vi "Autonomous Independent.vi"() -> ()   [LabVIEW 2013]
doc: "This VI is called when autonomous begins, and will automatically be terminated when autonomous ends. You can carry out timed or sensor driven robot movement independently without needing to return to the caller."
uses:
  <vilib>/Rock Robotics/WPI/Solenoid/WPI_SolenoidValue.ctl
  Robot Global Data.vi
  <vilib>/Rock Robotics/WPI/Solenoid/WPI_SolenoidSetEnum.vi
  <vilib>/Rock Robotics/WPI/RobotDrive/WPI_RobotDriveArcadeDrive_Standard(NoSaturation).vi
  <vilib>/Rock Robotics/WPI/RobotDrive/WPI_RobotDriveGetSetRefNum.vi
  <vilib>/Rock Robotics/WPI/Joystick/WPI_JoystickGetSetRefNum.vi
panel:
  in  "Current Shooter Status":T1(ring)=enum."Ready to fire"
  out "Timer for firing mech":dbl
  out "Hot?":bool
  out "Current Movement, for debugging":T2 {"Y Joystick Value" scale=1.0..-1.0; "X Joystick Value" scale=-1.0..1.0}
  in  "Array of robot movements":T3(array[cluster]) {"Y Joystick Value" scale=1.0..-1.0; "X Joystick Value" scale=-1.0..1.0}
  # "Be sure to right-click and choose Data Operations>>Make Current Value default if you want to save the array values with the VI"
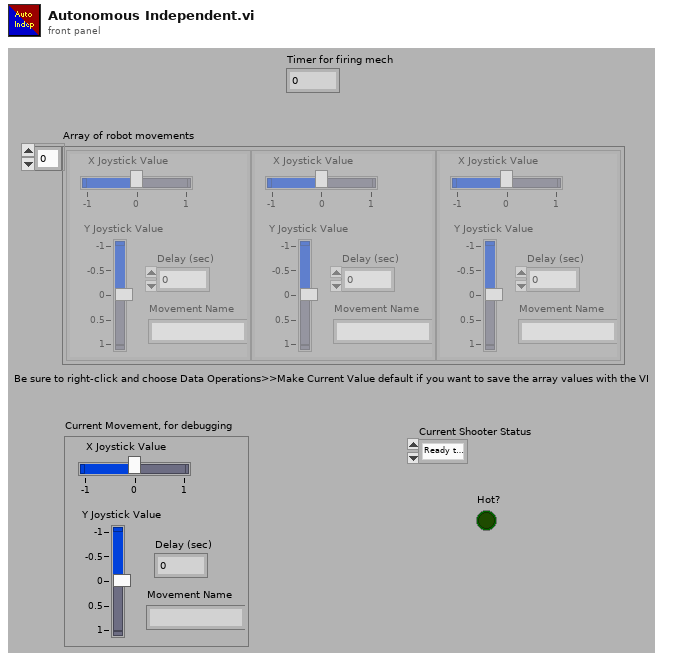
[diagram p1: front panel]
types:
  T1 = enum16{"Retracting", "Firing", "Ready to fire", "Pulling back", "Just fired"}
  T2 = cluster{"X Joystick Value":dbl, "Y Joystick Value":dbl, "Delay (sec)":dbl, "Movement Name":string}
  T3 = cluster{"X Joystick Value":dbl, "Y Joystick Value":dbl, "Delay (sec)":dbl, "Movement Name":string}[]
  T4 = typedef "WPI_JoystickDevRef.ctl" = cluster{"Device":T5}
  T5 = typedef "WPI_JoystickDeviceEnum.ctl" = enum16{"USB 1", "USB 2", "USB 3", "USB 4", "Kinect 1", "Kinect 2"}
  T6 = cluster{"axis 1 (x)":dbl, "axis 2 (y)":dbl, "axis 3 (throttle)":dbl, "axis 4":dbl, "axis 5":dbl, "axis 6":dbl}
  T7 = typedef "WPI_MotorControlDeviceRef.ctl" = cluster{"DeviceStatus":errorcluster, "Type":enum16{"PWM", "CAN"}, "PWM":cluster{"Digital Module":T8, "PWM Channel":T9, "DeadBand":T10}, "CAN":cluster{"Device Number":u8, "Control Mode":T11, "Semaphore":T12, "Max Vout":dbl}, "Invert":bool, "TransformRef":T13, "InvTransformRef":T13}
  T8 = typedef "FPGA_TypedefDigitalModule.ctl" = enum16{"Digital Module 1", "Digital Module 2"}
  T9 = typedef "FPGA_DIOPWMChannel.ctl" = enum8{"PWM 1", "PWM 2", "PWM 3", "PWM 4", "PWM 5", "PWM 6", "PWM 7", "PWM 8", "PWM 9", "PWM 10", "Invalid"}
  T10 = typedef "WPI_PWMDeadband.ctl" = cluster{"Name":string, "maxPositivePwm":i32, "minPositivePwm":i32, "centerPwm":i32, "maxNegativePwm":i32, "minNegativePwm":i32, "angularRange":u16}
  T11 = typedef "WPI_CANJaguar_ControlMode.ctl" = enum8{"Percent VBus", "Current", "Speed", "Position", "Voltage"}
  T12 = typedef "Semaphore RefNum" = refnum<k1>
  T13 = typedef "WPI_PWMTransform_ConPane.ctl" = refnum<vi>
  T14 = typedef "WPI_RobotDriveDevRef.ctl" = cluster{"DevStatus":errorcluster, "Motors[]":T7[], "Square Inputs":bool, "Max Output":dbl, "Isochronous":bool}
  T15 = typedef "WPI_EncoderDevRef.ctl" = cluster{"DevStatus":errorcluster, "EncoderIndex":T16, "CounterIndex":T17, "DistancePerCount":dbl, "Decoding Type":T18}
  T16 = typedef "FPGA_EncoderIdx.ctl" = enum8{"Enc 0", "Enc 1", "Enc 2", "Enc 3", "Invalid"}
  T17 = typedef "FPGA_CounterCtrSystemIndex.ctl" = enum8{"Ctr 0", "Ctr 1", "Ctr 2", "Ctr 3", "Ctr 4", "Ctr 5", "Ctr 6", "Ctr 7", "Invalid"}
  T18 = typedef "WPI_EncoderType.ctl" = enum16{"1x", "2x", "4x"}
  T19 = typedef "WPI_DigitalInputDevRef.ctl" = cluster{"DevStatus":errorcluster, "DIO Channel":T20, "Digital Module":T8}
  T20 = typedef "FPGA_DIOChannel.ctl" = enum8{"DIO 1", "DIO 2", "DIO 3", "DIO 4", "DIO 5", "DIO 6", "DIO 7", "DIO 8", "DIO 9", "DIO 10", "DIO 11", "DIO 12", "DIO 13", "DIO 14", "Invalid"}
  T21 = typedef "WPI_SolenoidValue.ctl" = enum16{"Off", "On", "Forward", "Reverse"}
  T22 = typedef "WPI_SolenoidDevRef.ctl" = cluster{"DevStatus":errorcluster, "Solenoid Module":T23, "Forward Solenoid Channel":T24, "Reverse Solenoid Channel":T24}
  T23 = typedef "FPGA_TypedefSolenoidModule.ctl" = enum16{"Solenoid Module 1", "Solenoid Module 2"}
  T24 = typedef "WPI_SolenoidChannel.ctl" = enum8{"Solenoid 1", "Solenoid 2", "Solenoid 3", "Solenoid 4", "Solenoid 5", "Solenoid 6", "Solenoid 7", "Solenoid 8", "Invalid"}
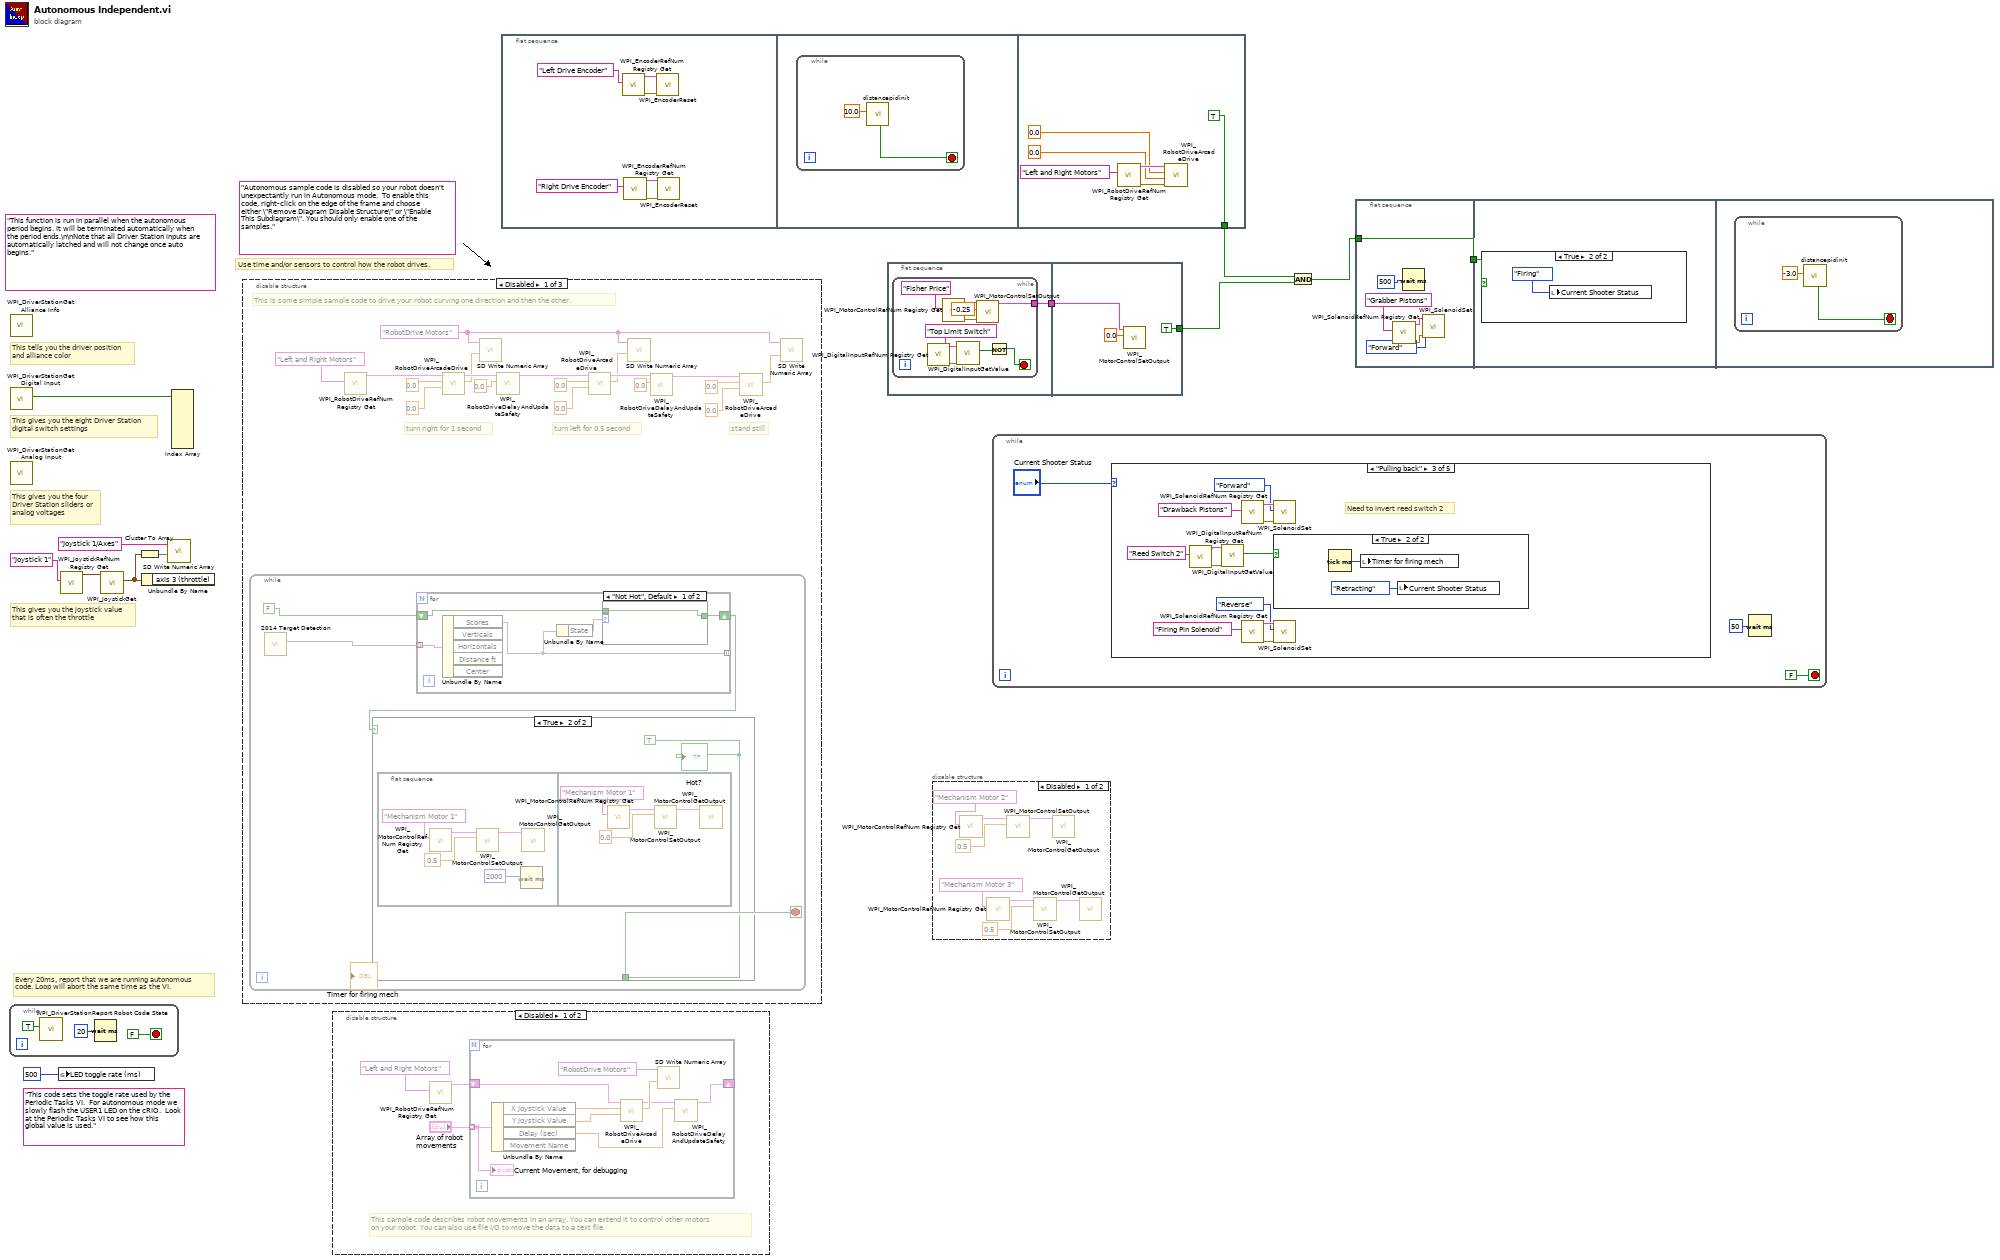
[diagram p0: block diagram]
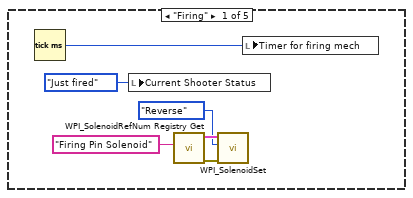
[diagram p3: hidden frame]
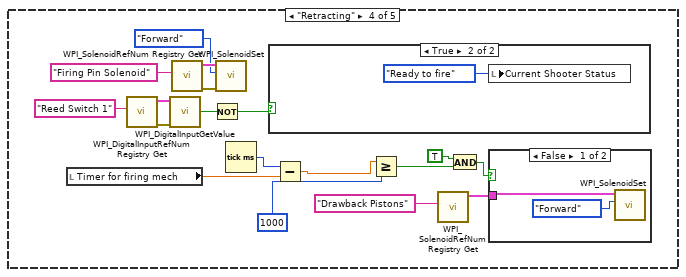
[diagram p6: hidden frame]
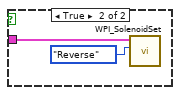
[diagram p8: hidden frame]
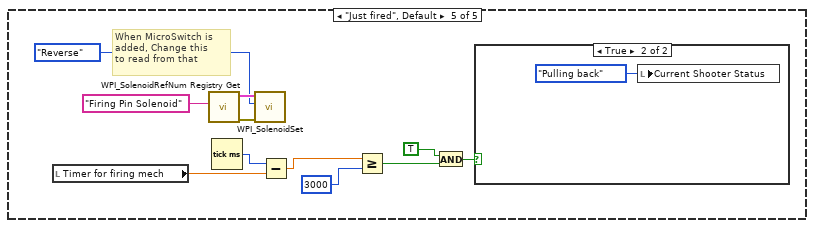
[diagram p9: hidden frame]
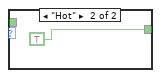
[diagram p13: hidden frame]
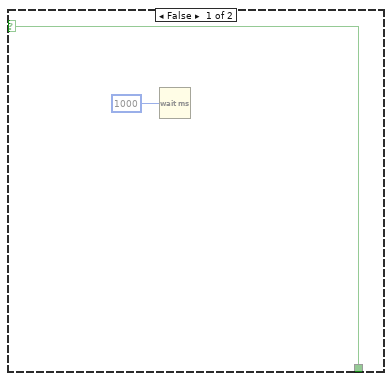
[diagram p14: hidden frame]
diagram:
  (unwired) "This code sets the toggle rate used by the Periodic Tasks VI.  For autonomous mode we slowly flash the USER1 LED on the cRIO.  Look at the Periodic Tasks VI to see how this global value is used."
  (unwired) "Autonomous sample code is disabled so your robot doesn't unexpectantly run in Autonomous mode.  To enable this code, right-click on the edge of the frame and choose either \"Remove Diagram Disable Structure\" or \"Enable This Subdiagram\". You should only enable one of the samples."
  (unwired) "This function is run in parallel when the autonomous period begins. It will be terminated automatically when the period ends.\n\nNote that all Driver Station inputs are automatically latched and will not change once auto begins."
  # "Every 20ms, report that we are running autonomous\ncode. Loop will abort the same time as the VI."
  # "This gives you the joystick value\nthat is often the throttle"
  # "Use time and/or sensors to control how the robot drives."
  # "This tells you the driver position\nand alliance color"
  # "This gives you the eight Driver Station\ndigital switch settings"
  # "This gives you the four\nDriver Station sliders or\nanalog voltages"
  n1 = while {
    stop <- FALSE stop-if-true
    n2 = call <vilib>:"WPI_DriverStationReport Robot Code State.vi"("Autonomous"=TRUE) -> ()  [unwired: 10 in, 1 out]
    n3 = Wait (ms)(milliseconds to wait=u32 20) -> ()  [unwired: 1 out]
  }
  n4 = call <vilib>:"WPI_DriverStationGet Alliance Info.vi"() -> ()  [unwired: 12 out]
  n5 = call <vilib>:"WPI_DriverStationGet Digital Input.vi"() -> ("Driver Station Digital Input (1-8)"=w12:bool[])  [unwired: 11 out]
  n6 = call <vilib>:"WPI_DriverStationGet Analog Input.vi"() -> ()  [unwired: 12 out]
  n7 = global write "Robot Global Data.vi" "LED toggle rate (ms)"(u32 500 ("LED ms toggle rate")) -> ()
  n8 = call <vilib>:"WPI_JoystickRefNum Registry Get.vi"("refnum name"="Joystick 1") -> ("JoystickDevRef"=w10:T4)  [unwired: 1 in, 9 out]
  n9 = call <vilib>:"WPI_JoystickGet.vi"("JoystickDevRef"=w10) -> ("Axes"=w7:T6)  [unwired: 1 in, 5 out]
  n10 = Cluster To Array(cluster=w7) -> (array=w8:dbl[])
  n11 = Unbundle By Name(w7) -> ()  [unwired: 1 out]
  n12 = call <vilib>:"SD Write Numeric Array.vi"("Numeric Array"=w8, "Name"="Joystick 1/Axes") -> ()  [unwired: 8 in, 2 out]
  n13 = Index Array(array=w12) -> ()  [unwired: 8 in, 8 out]
  n14 = disable-structure shown="Disabled" {
    frame Disabled {
      w16 = "RobotDrive Motors" ("Name")
      # "This is some simple sample code to drive your robot curving one direction and then the other."
      # "stand still"
      # "turn left for 0.5 second"
      # "turn right for 1 second"
      n15 = while {
        stop <- w37 stop-if-true
        n16 = call "2014 Target Detection.vi"() -> (2:w36)  [unwired: 11 in]
        n17 = for {
          tunnel: w36 -> [w42] mode=indexing
          tunnel: [w41] -> _ mode=indexing
          shift-right: [w39] -> w34
          shift-left: FALSE -> [w38]
          n18 = Unbundle By Name(w42) -> ("Scores"=w41)  [unwired: 4 out]
          n19 = Unbundle By Name(w41) -> ("State"=w40)
          n20 = case shown="\"Not Hot\", Default" w40 {
            tunnel: [w43 TRUE] -> w39
            tunnel: w38 -> [w43 _]
            frame "Not Hot", Default {
            }
            frame "Hot" {
            }
          }
        }
        n21 = case shown="True" w34 {
          selector: w34 -> [w45 _]
          tunnel: [w45 w47] -> w37
          frame False {
            n22 = Wait (ms)(milliseconds to wait=1000) -> ()  [unwired: 1 out]
          }
          frame True {
            w47 = TRUE
            n23 = flat-sequence {
              frame #0 {
                n24 = call <vilib>:"WPI_MotorControlRefNum Registry Get.vi"("refnum name"="Mechanism Motor 1") -> ("MotorControlDevRef"=w51:T7)  [unwired: 9 in, 1 out]
                n25 = call <vilib>:"WPI_MotorControlSetOutput.vi"("Output"=0.5, "MotorControlDevRef"=w51) -> ("MotorControlDevRef"=w49:T7)  [unwired: 7 in, 2 out]
                n26 = Wait (ms)(milliseconds to wait=2000) -> ()  [unwired: 1 out]
                n27 = call <vilib>:"WPI_MotorControlGetOutput.vi"("MotorControlDevRef"=w49) -> ()  [unwired: 8 in, 3 out]
              }
              frame #1 {
                n28 = call <vilib>:"WPI_MotorControlRefNum Registry Get.vi"("refnum name"="Mechanism Motor 1") -> ("MotorControlDevRef"=w55:T7)  [unwired: 9 in, 1 out]
                n29 = call <vilib>:"WPI_MotorControlSetOutput.vi"("Output"=0.0, "MotorControlDevRef"=w55) -> ("MotorControlDevRef"=w53:T7)  [unwired: 7 in, 2 out]
                n30 = call <vilib>:"WPI_MotorControlGetOutput.vi"("MotorControlDevRef"=w53) -> ()  [unwired: 8 in, 3 out]
              }
            }
            "Hot?" <- w47
          }
        }
      }
      n31 = call <vilib>:"WPI_RobotDriveRefNum Registry Get.vi"("refnum name"="Left and Right Motors") -> ("RobotDriveDevRef"=w20:T14)  [unwired: 1 in, 9 out]
      n32 = call-poly <vilib>:"WPI_RobotDriveArcadeDrive.vi"("Y axis value"=0.0 ("X axis value"), "X axis value"=0.0, "RobotDriveDevRef"=w20) -> ("Motor Values"=w19:dbl[], "RobotDriveDevRef"=w27:T14)  [unwired: 1 in, 6 out]
      n33 = call <vilib>:"SD Write Numeric Array.vi"("Numeric Array"=w19, "Name"=w16) -> ()  [unwired: 8 in, 2 out]
      n34 = call <vilib>:"WPI_RobotDriveDelayAndUpdateSafety.vi"("Delay (s)"=0.0, "RobotDriveDevRef"=w27) -> ("RobotDriveDevRef 2"=w26:T14)  [unwired: 8 in, 1 out]
      n35 = call-poly <vilib>:"WPI_RobotDriveArcadeDrive.vi"("Y axis value"=0.0 ("X axis value"), "X axis value"=0.0, "RobotDriveDevRef"=w26) -> ("Motor Values"=w18:dbl[], "RobotDriveDevRef"=w25:T14)  [unwired: 1 in, 6 out]
      n36 = call <vilib>:"SD Write Numeric Array.vi"("Numeric Array"=w18, "Name"=w16) -> ()  [unwired: 8 in, 2 out]
      n37 = call <vilib>:"WPI_RobotDriveDelayAndUpdateSafety.vi"("Delay (s)"=0.0, "RobotDriveDevRef"=w25) -> ("RobotDriveDevRef 2"=w24:T14)  [unwired: 8 in, 1 out]
      n38 = call-poly <vilib>:"WPI_RobotDriveArcadeDrive.vi"("Y axis value"=0.0 ("X axis value"), "X axis value"=0.0, "RobotDriveDevRef"=w24) -> ("Motor Values"=w17:dbl[])  [unwired: 1 in, 7 out]
      n39 = call <vilib>:"SD Write Numeric Array.vi"("Numeric Array"=w17, "Name"=w16) -> ()  [unwired: 8 in, 2 out]
    }
    frame Disabled {
    }
    frame Enabled {
    }
  }
  n40 = disable-structure shown="Disabled" {
    frame Disabled {
      # "This sample code describes robot movements in an array. You can extend it to control other motors\non your robot. You can also use file I/O to move the data to a text file."
      n41 = call <vilib>:"WPI_RobotDriveRefNum Registry Get.vi"("refnum name"="Left and Right Motors") -> ("RobotDriveDevRef"=w58:T14)  [unwired: 1 in, 9 out]
      n42 = for {
        shift-right: [w64] -> _
        shift-left: w58 -> [w65]
        tunnel: "Array of robot movements" -> [w60] mode=indexing
        n43 = Unbundle By Name(w60) -> ("X Joystick Value"=w63:dbl, "Y Joystick Value"=w62:dbl, "Delay (sec)"=w61:dbl)  [unwired: 1 out]
        n44 = call-poly <vilib>:"WPI_RobotDriveArcadeDrive.vi"("Y axis value"=w62, "X axis value"=w63, "RobotDriveDevRef"=w65) -> ("Motor Values"=w67:dbl[], "RobotDriveDevRef"=w66:T14)  [unwired: 1 in, 6 out]
        n45 = call <vilib>:"SD Write Numeric Array.vi"("Numeric Array"=w67, "Name"="RobotDrive Motors") -> ()  [unwired: 8 in, 2 out]
        n46 = call <vilib>:"WPI_RobotDriveDelayAndUpdateSafety.vi"("Delay (s)"=w61, "RobotDriveDevRef"=w66) -> ("RobotDriveDevRef 2"=w64:T14)  [unwired: 8 in, 1 out]
        "Current Movement, for debugging" <- w60
      }
    }
    frame Enabled {
    }
  }
  n47 = flat-sequence {
    tunnel: [TRUE] -> w2
    frame #0 {
      n48 = call <vilib>:"WPI_EncoderRefNum Registry Get.vi"("refnum name"="Left Drive Encoder") -> ("error out"=w72:errorcluster, "EncoderDevRef"=w71:T15)  [unwired: 9 in]
      n49 = call <vilib>:"WPI_EncoderRefNum Registry Get.vi"("refnum name"="Right Drive Encoder") -> ("error out"=w70:errorcluster, "EncoderDevRef"=w69:T15)  [unwired: 9 in]
      n50 = call <vilib>:"WPI_EncoderReset.vi"("error in (no error)"=w72, "EncoderDevRef"=w71) -> ()  [unwired: 8 in, 2 out]
      n51 = call <vilib>:"WPI_EncoderReset.vi"("error in (no error)"=w70, "EncoderDevRef"=w69) -> ()  [unwired: 8 in, 2 out]
    }
    frame #1 {
      n52 = while {
        stop <- w75 stop-if-true
        n53 = call "distancepidinit.vi"("Distance From Target"=10.0) -> ("Done?"=w75:bool)  [unwired: 10 in]
      }
    }
    frame #2 {
      n54 = call <vilib>:"WPI_RobotDriveRefNum Registry Get.vi"("refnum name"="Left and Right Motors") -> ("error out"=w82:errorcluster, "RobotDriveDevRef"=w81:T14)  [unwired: 9 in]
      n55 = call-poly <vilib>:"WPI_RobotDriveArcadeDrive.vi"("error in (no error)"=w82, "Y axis value"=0.0, "X axis value"=0.0, "RobotDriveDevRef"=w81) -> ()  [unwired: 5 in, 3 out]
    }
  }
  n56 = flat-sequence {
    tunnel: [w83] -> w5
    tunnel: w5 -> [w95]
    tunnel: [TRUE] -> w1
    frame #0 {
      n57 = while {
        tunnel: [w89] -> w83
        stop <- w84 stop-if-true
        n58 = call <vilib>:"WPI_DigitalInputRefNum Registry Get.vi"("refnum name"="Top Limit Switch") -> ("error out"=w86:errorcluster, "DigitalInputDevRef"=w87:T19)  [unwired: 9 in]
        n59 = call <vilib>:"WPI_MotorControlRefNum Registry Get.vi"("refnum name"="Fisher Price") -> ("error out"=w92:errorcluster, "MotorControlDevRef"=w91:T7)  [unwired: 9 in]
        n60 = call <vilib>:"WPI_DigitalInputGetValue.vi"("error in (no error)"=w86, "DigitalInputDevRef"=w87) -> ("Value"=w85:bool)  [unwired: 7 in, 2 out]
        n61 = call <vilib>:"WPI_MotorControlSetOutput.vi"("error in (no error)"=w92, "Output"=-0.25, "MotorControlDevRef"=w91) -> ("MotorControlDevRef"=w89:T7)  [unwired: 6 in, 2 out]
        n62 = Not(x=w85) -> (.not. x?=w84:bool)
      }
    }
    frame #1 {
      n63 = call <vilib>:"WPI_MotorControlSetOutput.vi"("Output"=0.0, "MotorControlDevRef"=w95) -> ()  [unwired: 7 in, 3 out]
    }
  }
  n64 = disable-structure shown="Disabled" {
    frame Disabled {
      n65 = call <vilib>:"WPI_MotorControlRefNum Registry Get.vi"("refnum name"="Mechanism Motor 2") -> ("MotorControlDevRef"=w104:T7)  [unwired: 9 in, 1 out]
      n66 = call <vilib>:"WPI_MotorControlRefNum Registry Get.vi"("refnum name"="Mechanism Motor 3") -> ("MotorControlDevRef"=w99:T7)  [unwired: 9 in, 1 out]
      n67 = call <vilib>:"WPI_MotorControlSetOutput.vi"("Output"=0.5, "MotorControlDevRef"=w104) -> ("MotorControlDevRef"=w102:T7)  [unwired: 7 in, 2 out]
      n68 = call <vilib>:"WPI_MotorControlSetOutput.vi"("Output"=0.5, "MotorControlDevRef"=w99) -> ("MotorControlDevRef"=w97:T7)  [unwired: 7 in, 2 out]
      n69 = call <vilib>:"WPI_MotorControlGetOutput.vi"("MotorControlDevRef"=w102) -> ()  [unwired: 8 in, 3 out]
      n70 = call <vilib>:"WPI_MotorControlGetOutput.vi"("MotorControlDevRef"=w97) -> ()  [unwired: 8 in, 3 out]
    }
    frame Enabled {
    }
  }
  n71 = while {
    stop <- FALSE stop-if-true
    n72 = case shown="\"Pulling back\"" "Current Shooter Status" {
      frame "Firing" {
        n73 = Tick Count (ms)() -> (millisecond timer value=w108:u32)
        n74 = local write "Current Shooter Status"(T1."Just fired" ("Current Shooter Status")) -> ()
        n75 = call <vilib>:"WPI_SolenoidRefNum Registry Get.vi"("refnum name"="Firing Pin Solenoid") -> ("error out"=w112:errorcluster, "SolenoidDevRef"=w111:T22)  [unwired: 9 in]
        n76 = call-poly <vilib>:"WPI_SolenoidSet.vi"("error in (no error)"=w112, "Value"=WPI_SolenoidValue."Reverse", "SolenoidDevRef"=w111) -> ()  [unwired: 7 in, 2 out]
        n77 = local write "Timer for firing mech"(w108) -> ()
      }
      frame "Ready to fire" {
      }
      frame "Pulling back" {
        # "Need to invert reed switch 2"
        n78 = call <vilib>:"WPI_DigitalInputRefNum Registry Get.vi"("refnum name"="Reed Switch 2") -> ("error out"=w115:errorcluster, "DigitalInputDevRef"=w116:T19)  [unwired: 9 in]
        n79 = call <vilib>:"WPI_DigitalInputGetValue.vi"("error in (no error)"=w115, "DigitalInputDevRef"=w116) -> ("Value"=w114:bool)  [unwired: 7 in, 2 out]
        n80 = call <vilib>:"WPI_SolenoidRefNum Registry Get.vi"("refnum name"="Drawback Pistons") -> ("error out"=w120:errorcluster, "SolenoidDevRef"=w119:T22)  [unwired: 9 in]
        n81 = call <vilib>:"WPI_SolenoidRefNum Registry Get.vi"("refnum name"="Firing Pin Solenoid") -> ("error out"=w124:errorcluster, "SolenoidDevRef"=w123:T22)  [unwired: 9 in]
        n82 = call-poly <vilib>:"WPI_SolenoidSet.vi"("error in (no error)"=w120, "Value"=WPI_SolenoidValue."Forward", "SolenoidDevRef"=w119) -> ()  [unwired: 7 in, 2 out]
        n83 = case shown="True" w114 {
          frame False {
          }
          frame True {
            n84 = Tick Count (ms)() -> (millisecond timer value=w126:u32)
            n85 = local write "Timer for firing mech"(w126) -> ()
            n86 = local write "Current Shooter Status"(T1."Retracting" ("Current Shooter Status")) -> ()
          }
        }
        n87 = call-poly <vilib>:"WPI_SolenoidSet.vi"("error in (no error)"=w124, "Value"=WPI_SolenoidValue."Reverse", "SolenoidDevRef"=w123) -> ()  [unwired: 7 in, 2 out]
      }
      frame "Retracting" {
        n88 = local read "Timer for firing mech"() -> (w141:dbl)
        n89 = call <vilib>:"WPI_DigitalInputRefNum Registry Get.vi"("refnum name"="Reed Switch 1") -> ("error out"=w135:errorcluster, "DigitalInputDevRef"=w136:T19)  [unwired: 9 in]
        n90 = call <vilib>:"WPI_DigitalInputGetValue.vi"("error in (no error)"=w135, "DigitalInputDevRef"=w136) -> ("Value"=w128:bool)  [unwired: 7 in, 2 out]
        n91 = call <vilib>:"WPI_SolenoidRefNum Registry Get.vi"("refnum name"="Firing Pin Solenoid") -> ("error out"=w144:errorcluster, "SolenoidDevRef"=w143:T22)  [unwired: 9 in]
        n92 = Not(x=w128) -> (.not. x?=w129:bool)
        n93 = call-poly <vilib>:"WPI_SolenoidSet.vi"("error in (no error)"=w144, "Value"=WPI_SolenoidValue."Forward", "SolenoidDevRef"=w143) -> ()  [unwired: 7 in, 2 out]
        n94 = Tick Count (ms)() -> (millisecond timer value=w140:u32)
        n95 = case shown="True" w129 {
          frame False {
          }
          frame True {
            n96 = local write "Current Shooter Status"(T1."Ready to fire" ("Current Shooter Status")) -> ()
          }
        }
        n97 = Subtract(x=w140, y=w141) -> (x-y=w131:dbl)
        n98 = Greater Or Equal?(x=w131, y=1000) -> (x >= y?=w133:bool)
        n99 = call <vilib>:"WPI_SolenoidRefNum Registry Get.vi"("refnum name"="Drawback Pistons") -> ("SolenoidDevRef"=w138:T22)  [unwired: 9 in, 1 out]
        n100 = And(x=TRUE, y=w133) -> (x .and. y?=w134:bool)
        n101 = case shown="False" w134 {
          tunnel: w138 -> [w147 w149]
          frame False {
            n102 = call-poly <vilib>:"WPI_SolenoidSet.vi"("Value"=WPI_SolenoidValue."Forward", "SolenoidDevRef"=w147) -> ()  [unwired: 8 in, 2 out]
          }
          frame True {
            n103 = call-poly <vilib>:"WPI_SolenoidSet.vi"("Value"=WPI_SolenoidValue."Reverse", "SolenoidDevRef"=w149) -> ()  [unwired: 8 in, 2 out]
          }
        }
      }
      frame "Just fired", Default {
        # "When MicroSwitch is \nadded, Change this \nto read from that"
        n104 = local read "Timer for firing mech"() -> (w161:dbl)
        n105 = call <vilib>:"WPI_SolenoidRefNum Registry Get.vi"("refnum name"="Firing Pin Solenoid") -> ("error out"=w158:errorcluster, "SolenoidDevRef"=w157:T22)  [unwired: 9 in]
        n106 = Tick Count (ms)() -> (millisecond timer value=w160:u32)
        n107 = call-poly <vilib>:"WPI_SolenoidSet.vi"("error in (no error)"=w158, "Value"=WPI_SolenoidValue."Reverse", "SolenoidDevRef"=w157) -> ()  [unwired: 7 in, 2 out]
        n108 = Subtract(x=w160, y=w161) -> (x-y=w152:dbl)
        n109 = Greater Or Equal?(x=w152, y=3000) -> (x >= y?=w155:bool)
        n110 = And(x=TRUE, y=w155) -> (x .and. y?=w154:bool)
        n111 = case shown="True" w154 {
          frame False {
          }
          frame True {
            n112 = local write "Current Shooter Status"(T1."Pulling back" ("Current Shooter Status")) -> ()
          }
        }
      }
    }
    n113 = Wait (ms)(milliseconds to wait=u32 50) -> ()  [unwired: 1 out]
  }
  n114 = And(x=w2, y=w1) -> (x .and. y?=w4:bool)
  n115 = flat-sequence {
    tunnel: [w168] -> w3
    tunnel: w4 -> [w168]
    tunnel: w3 -> [w169]
    frame #0 {
      n116 = call <vilib>:"WPI_SolenoidRefNum Registry Get.vi"("refnum name"="Grabber Pistons") -> ("error out"=w165:errorcluster, "SolenoidDevRef"=w164:T22)  [unwired: 9 in]
      n117 = Wait (ms)(milliseconds to wait=u32 500) -> ()  [unwired: 1 out]
      n118 = call-poly <vilib>:"WPI_SolenoidSet.vi"("error in (no error)"=w165, "Value"=WPI_SolenoidValue."Forward", "SolenoidDevRef"=w164) -> ()  [unwired: 7 in, 2 out]
    }
    frame #1 {
      n119 = case shown="True" w169 {
        frame False {
        }
        frame True {
          n120 = local write "Current Shooter Status"(T1."Firing" ("Current Shooter Status")) -> ()
        }
      }
    }
    frame #2 {
      n121 = while {
        stop <- w171 stop-if-true
        n122 = call "distancepidinit.vi"("Distance From Target"=-3.0) -> ("Done?"=w171:bool)  [unwired: 10 in]
      }
    }
  }
